vi "Get Classes Names.vi"(8 "error in (no error)":errorcluster) -> (0 "error out":errorcluster, 3 "Classes Names":string[](array[string]))   [LabVIEW 2020, in "Oscilloscope VI.lvlib"]
uses:
  Oscilloscope VI/Oscilloscope VI.lvlib
  Oscilloscope.lvclass
  Scope 1 Test/Scope 1 Test.lvclass
  C:/Users/DELL/Documents/GitClones/Labview/OscilloscopeDQMH_OOP/Oscilloscope_DQMH_OOP/Libraries/Classes/Oscilloscope/Oscilloscope.lvclass
  Scope 2 Test/Scope 2 Test.lvclass
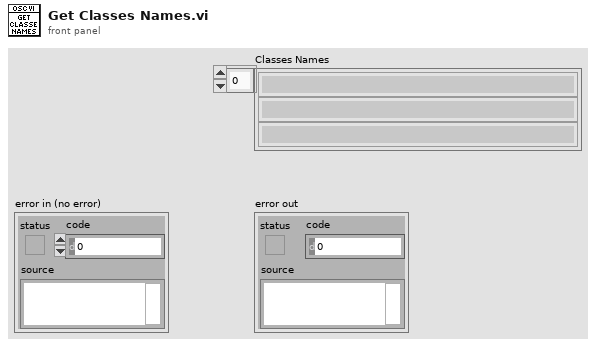
[diagram p1: front panel]
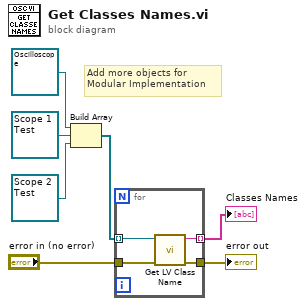
[diagram p0: block diagram]
diagram:
  # "Add more objects for\nModular Implementation"
  n1 = Build Array(refnum<class "Oscilloscope.lvclass"> refnum ("Oscilloscope VI.lvlib:Oscilloscope.lvclass"), refnum<class "Scope 1 Test.lvclass"> refnum ("Oscilloscope VI.lvlib:Scope 1 Test.lvclass"), refnum<class "Scope 2 Test.lvclass"> refnum ("Oscilloscope VI.lvlib:Scope 2 Test.lvclass")) -> (w6:refnum<class "Oscilloscope.lvclass">[])
  n2 = for {
    tunnel: w6 -> [w11] mode=indexing
    tunnel: [w10] -> w5 mode=indexing
    tunnel: "error in (no error)" -> [w9]
    tunnel: [w8] -> w3
    n3 = call <vilib>:"Get LV Class Name.vi"("error in (no error)"=w9, "object"=w11) -> ("error out"=w8:errorcluster, "class name"=w10:string)  [unwired: 8 in]
  }
  "Classes Names" <- w5
  "error out" <- w3
